vi "Dash LEd Control.vi"(10 "Vehicle Status":T2) -> (1 "Red LED":T1, 2 "Yellow LED":T1, 3 "Green LED":T1)   [LabVIEW 2014]
uses:
  Vehicle Status/Subsystem Status.ctl
  Vehicle Status/Subsystem Status Severity.ctl
  Vehicle Status/Subsystem Status Message.ctl
  Dash LED Status.ctl
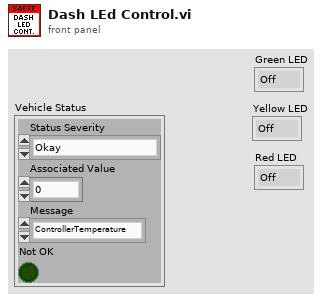
[diagram p1: front panel]
types:
  T1 = typedef "Dash LED Status.ctl" = enum16{"Off", "Flashing", "On"}
  T2 = typedef "Subsystem Status.ctl" = cluster{"Status Severity":T3, "Associated Value":sgl, "Message":T4, "Not OK":bool}
  T3 = typedef "Subsystem Status Severity.ctl" = enum16{"Okay", "Short Warning", "Long Warning", "Return to Pits", "Error", "Danger"}
  T4 = typedef "Subsystem Status Message.ctl" = enum16{"ControllerTemperature", "MotorTemperature", "BatteryTemperature", "BatteryLowVoltage", "LVBattery", "sbRIOTemperature", "Precharge", "BSPD", "IMD", "RemoteReturnToPits", "EStopInterrupted", "NoCellComms", "MCOverSpeed", "MCOverCurrent", "MCOverVoltage", "MCInverterOverTemp", "MCDirectionCommand", "MCInverterTimeout", "MCDesatFault", "MCHWOverCurrent", "MCUnderVoltage", "MCCommandMessageLost", "MotorOverTemp", "MCModAOverTemp", "MCModBOverTemp", "MCModCOverTemp", "MCPCBOverTemp", "MCGateDrv1OverTemp", "MCDateDrv2OverTemp", "MCCurrentSensorFault", "MCResolverNotConnected", "ShutdownLatchTripped", "UnknownBMS", "RemoteEmergency"}
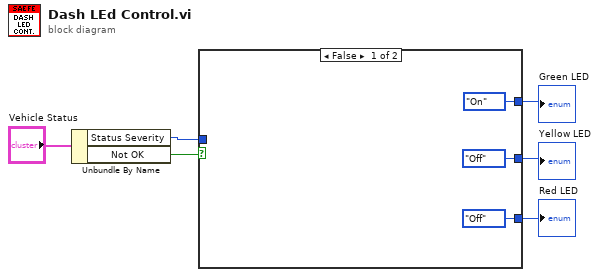
[diagram p0: block diagram]
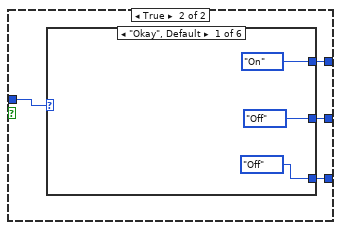
[diagram p2: hidden frame]
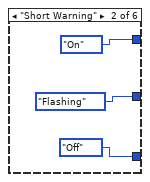
[diagram p3: hidden frame]
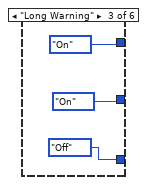
[diagram p4: hidden frame]
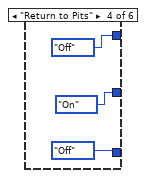
[diagram p5: hidden frame]
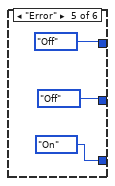
[diagram p6: hidden frame]
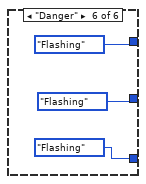
[diagram p7: hidden frame]
diagram:
  n1 = Unbundle By Name("Vehicle Status") -> ("Status Severity"=w2:T3, "Not OK"=w1:bool)
  n2 = case shown="False" w1 {
    tunnel: [Dash_LED_Status."On" ("Green LED") w13] -> w6
    tunnel: [Dash_LED_Status."Off" ("Green LED") w12] -> w5
    tunnel: [Dash_LED_Status."Off" ("Green LED") w11] -> w4
    tunnel: w2 -> [_ w10]
    frame False {
    }
    frame True {
      n3 = case shown="\"Okay\", Default" w10 {
        tunnel: [Dash_LED_Status."On" ("Green LED") Dash_LED_Status."On" ("Green LED") Dash_LED_Status."On" ("Green LED") Dash_LED_Status."Off" ("Green LED") Dash_LED_Status."Off" ("Green LED") Dash_LED_Status."Flashing" ("Green LED")] -> w13
        tunnel: [Dash_LED_Status."Off" ("Green LED") Dash_LED_Status."Flashing" ("Green LED") Dash_LED_Status."On" ("Green LED") Dash_LED_Status."On" ("Green LED") Dash_LED_Status."Off" ("Green LED") Dash_LED_Status."Flashing" ("Green LED")] -> w12
        tunnel: [Dash_LED_Status."Off" ("Green LED") Dash_LED_Status."Off" ("Green LED") Dash_LED_Status."Off" ("Green LED") Dash_LED_Status."Off" ("Green LED") Dash_LED_Status."On" ("Green LED") Dash_LED_Status."Flashing" ("Green LED")] -> w11
        frame "Okay", Default {
        }
        frame "Short Warning" {
        }
        frame "Long Warning" {
        }
        frame "Return to Pits" {
        }
        frame "Error" {
        }
        frame "Danger" {
        }
      }
    }
  }
  "Green LED" <- w6
  "Yellow LED" <- w5
  "Red LED" <- w4
